vi "Set Listbox ref.vi"(8 "error in (no error)":errorcluster, 11 "ListRef":refnum<vi>) -> (0 "error out":errorcluster)   [LabVIEW 2019]
uses:
  <vilib>/picture/picture.llb/Draw True-Color Pixmap.vi
panel:
  in  "stop":bool
  in  "Symbols":T1(array[cluster])
  in  "ProcessList":i32(listbox) caption="動作流程"
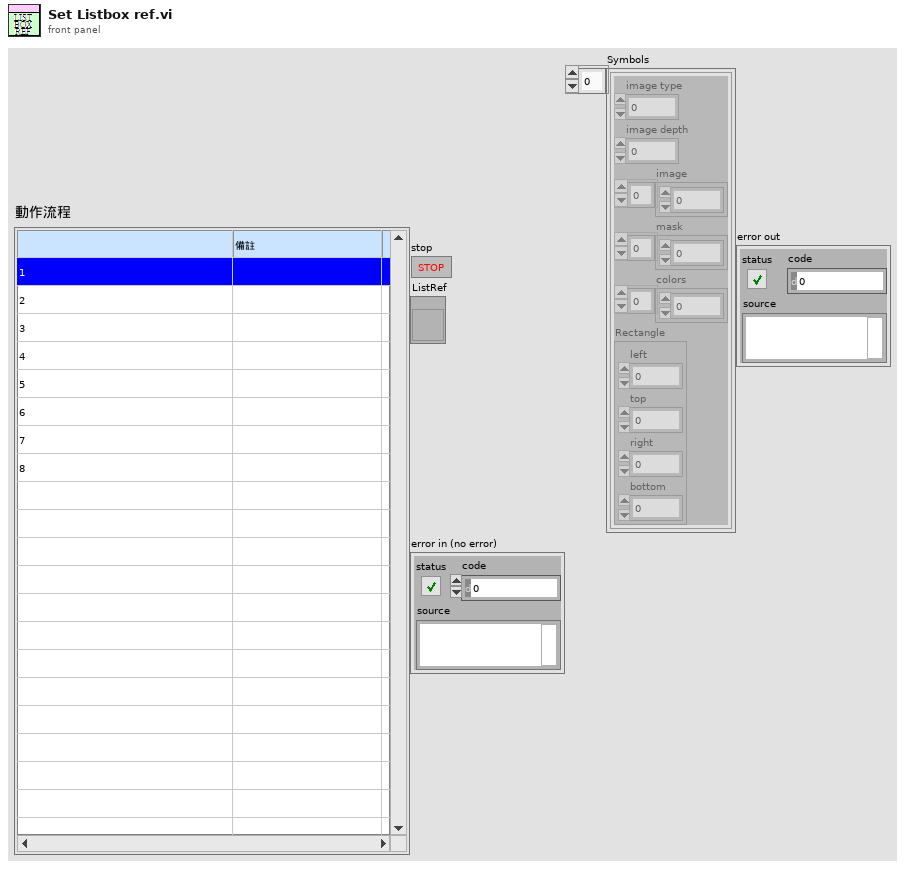
[diagram p1: front panel]
types:
  T1 = cluster{"image type":i32, "image depth":i32, "image":u8[], "mask":u8[], "colors":u32[], "Rectangle":cluster{"left":i16, "top":i16, "right":i16, "bottom":i16}}[]
  T2 = cluster{"left":i16, "top":i16, "right":i16, "bottom":i16}
  T3 = cluster{"Width":u16, "Style":enum32{"Solid", "Dash", "Dot", "DashDot", "DashDotDot"}}
  T4 = typedef "imagedata.ctl" = cluster{"image type":i32, "image depth":i32, "image":u8[], "mask":u8[], "colors":u32[], "Rectangle":cluster{"left":i16, "top":i16, "right":i16, "bottom":i16}}
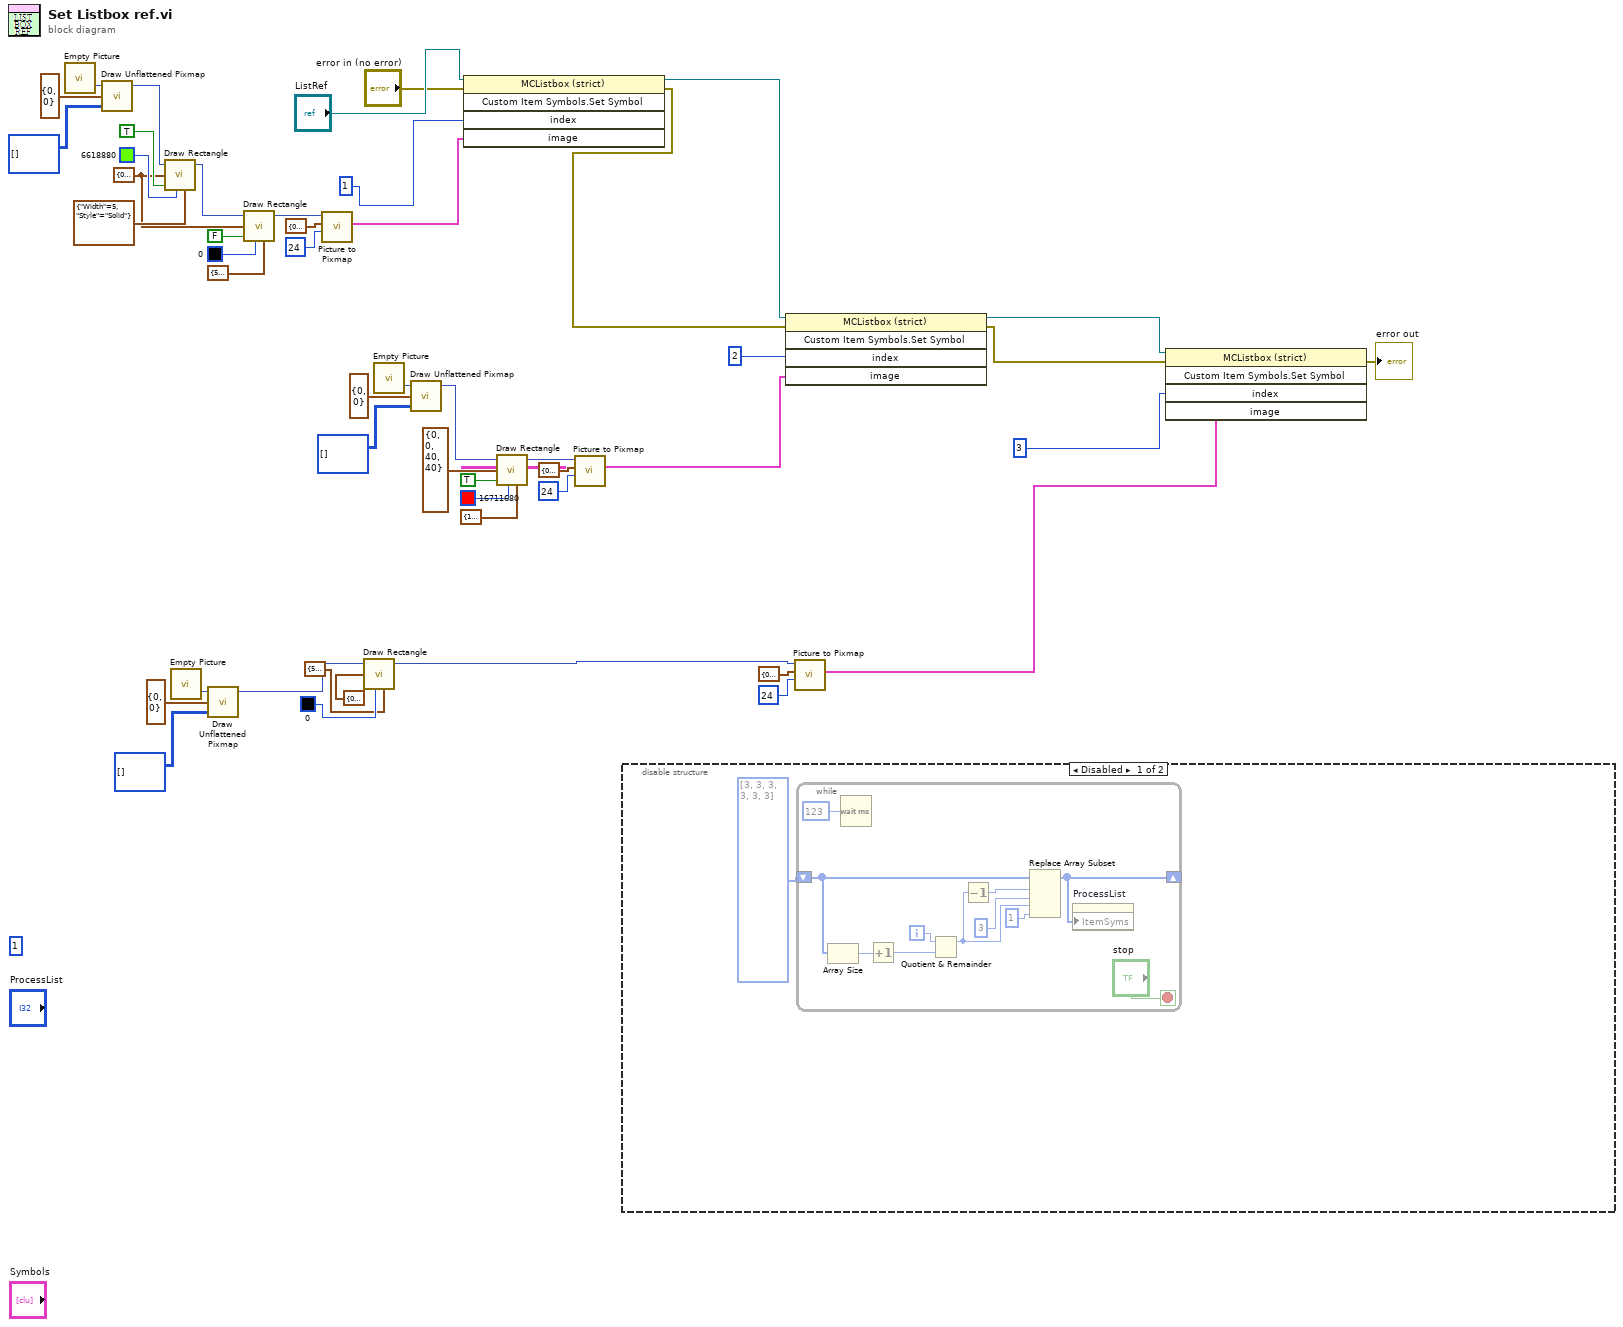
[diagram p0: block diagram]
diagram:
  (unwired) 1 ("Index")
  w19 = T2 {"left"=0, "top"=0, "right"=40, "bottom"=40} ("rect")
  n1 = call "Empty Picture"() -> ("empty picture"=w49:picture)
  n2 = call-poly <vilib>:"Draw Unflattened Pixmap.vi"("picture"=w49, "top left point(0, 0)"=cluster{"x":i16, "y":i16} {"x"=0, "y"=0}, "data (RGB format)"=u32[][] []) -> ("new picture"=w30:picture)  [unwired: 6 in]
  n3 = call <vilib>:"Draw Rectangle.vi"("picture"=w30, "rect"=w19, "fill?(F)"=TRUE, "color(black)"=u32 6618880, "pen"=T3 {"Width"=5, "Style"=enum."Solid"}) -> ("new picture"=w29:picture)  [unwired: 4 in]
  n4 = call "Empty Picture"() -> ("empty picture"=w22:picture)
  n5 = call-poly <vilib>:"Draw Unflattened Pixmap.vi"("picture"=w22, "top left point(0, 0)"=cluster{"x":i16, "y":i16} {"x"=0, "y"=0}, "data (RGB format)"=u32[][] []) -> ("new picture"=w20:picture)  [unwired: 6 in]
  n6 = call <vilib>:"Draw Rectangle.vi"("picture"=w29, "rect"=w19, "fill?(F)"=FALSE, "color(black)"=u32 0, "pen"=T3 {"Width"=5, "Style"=enum."Solid"}) -> ("new picture"=w44:picture)  [unwired: 4 in]
  n7 = call <vilib>:"Picture to Pixmap.vi"("depth"=24, "rect"=T2 {"left"=0, "top"=0, "right"=40, "bottom"=40}, "picture"=w44) -> ("image data"=w12:T4)  [unwired: 7 in, 1 out]
  n8 = call <vilib>:"Draw Rectangle.vi"("picture"=w20, "rect"=T2 {"left"=0, "top"=0, "right"=40, "bottom"=40}, "color(black)"=u32 0, "pen"=T3 {"Width"=5, "Style"=enum."Solid"}) -> ("new picture"=w17:picture)  [unwired: 5 in]
  n9 = call "Empty Picture"() -> ("empty picture"=w31:picture)
  n10 = call-poly <vilib>:"Draw Unflattened Pixmap.vi"("picture"=w31, "top left point(0, 0)"=cluster{"x":i16, "y":i16} {"x"=0, "y"=0}, "data (RGB format)"=u32[][] []) -> ("new picture"=w36:picture)  [unwired: 6 in]
  n11 = invoke class="MCListbox (strict)" method="Custom Item Symbols.Set Symbol"(reference="ListRef", error in="error in (no error)", "index"=1 ("Index"), "image"=w12) -> (reference out=w11:refnum<vi>, error out=w9:errorcluster)  [unwired: 1 in, 3 out]
  n12 = call <vilib>:"Draw Rectangle.vi"("picture"=w36, "rect"=T2 {"left"=0, "top"=0, "right"=40, "bottom"=40}, "fill?(F)"=TRUE, "color(black)"=u32 16711680, "pen"=T3 {"Width"=10, "Style"=enum."Solid"}) -> ("new picture"=w37:picture)  [unwired: 4 in]
  n13 = call <vilib>:"Picture to Pixmap.vi"("depth"=24, "rect"=T2 {"left"=0, "top"=0, "right"=40, "bottom"=40}, "picture"=w37) -> ("image data"=w8:T4)  [unwired: 7 in, 1 out]
  n14 = disable-structure shown="Disabled" {
    frame Disabled {
      n15 = while {
        shift-right: [w58] -> _
        shift-left: i32[] [3, 3, 3, 3, 3, 3] ("Item Symbols") -> [w59]
        i -> [w61]
        stop <- "stop" stop-if-true
        n16 = Array Size(array=w59) -> (size(s)=w60:i32)
        n17 = Wait (ms)(milliseconds to wait=u32 123) -> ()  [unwired: 1 out]
        n18 = Increment(x=w60) -> (x+1=w51:i32)
        n19 = Quotient & Remainder(x=w61, y=w51) -> (x-y*floor(x/y)=w55:i32)  [unwired: 1 out]
        n20 = Decrement(x=w55) -> (x-1=w57:i32)
        n21 = Replace Array Subset(array=w59, new element #1=3 ("new element/subarray"), index #1=w57, new element #2=1 ("new element/subarray"), index #2=w55) -> (w58:i32[])
        n22 = property on="ProcessList" class="MCListbox (strict)"("ItemSyms"=w58) -> ()  [unwired: 2 in, 2 out]
      }
    }
    frame Enabled {
    }
  }
  n23 = invoke class="MCListbox (strict)" method="Custom Item Symbols.Set Symbol"(reference=w11, error in=w9, "index"=2 ("Index"), "image"=w8) -> (reference out=w7:refnum<vi>, error out=w4:errorcluster)  [unwired: 1 in, 3 out]
  n24 = call <vilib>:"Picture to Pixmap.vi"("depth"=24, "rect"=T2 {"left"=0, "top"=0, "right"=40, "bottom"=40}, "picture"=w17) -> ("image data"=w5:T4)  [unwired: 7 in, 1 out]
  n25 = invoke class="MCListbox (strict)" method="Custom Item Symbols.Set Symbol"(reference=w7, error in=w4, "index"=3 ("Index"), "image"=w5) -> (error out=→"error out":errorcluster)  [unwired: 1 in, 4 out]
